vi "Get Properties by Class ID.vi"(8 "error in (no error)":errorcluster, 11 "Class ID":string) -> (0 "error out":errorcluster, 3 "Properties[]":T1(array[cluster]))   [LabVIEW 2023]
doc: "<b> </b> <b> </b>\n© 2017 Q Software Innovations, LLC\nwritten by Quentin \"Q\" Alldredge\nproduced in LabVIEW 2015\n\nsupport@qsoftwareinnovations.com\nwww.qsoftwareinnovations.com\n\nAll rights reserved.\n\nRedistribution and use in source and binary forms, with or without modification, are permitted provided that the following conditions are met:\n\n * Redistributions of source code must retain the above copyright notice, this list of conditions and the following disclaimer.\n * Redistributions in binary form must reproduce the above copyright notice, this list of conditions and the following disclaimer in the documentation and/or other materials provided with the distribution.\n * Neither the name of Q Software Innovations, LLC. nor the names of its contributors may be used to endorse or promote products derived from this software without specific prior written permission.\n\nTHIS SOFTWARE IS PROVIDED BY THE COPYRIGHT HOLDERS AND CONTRIBUTORS \"AS IS\" AND ANY EXPRESS OR IMPLIED WARRANTIES, INCLUDING, BUT NOT LIMITED TO, THE IMPLIED WARRANTIES OF MERCHANTABILITY AND FITNESS FOR A PARTICULAR PURPOSE ARE DISCLAIMED. IN NO EVENT SHALL THE COPYRIGHT OWNER OR CONTRIBUTORS BE LIABLE FOR ANY DIRECT, INDIRECT, INCIDENTAL, SPECIAL, EXEMPLARY, OR CONSEQUENTIAL DAMAGES (INCLUDING, BUT NOT LIMITED TO, PROCUREMENT OF SUBSTITUTE GOODS OR SERVICES; LOSS OF USE, DATA, OR PROFITS; OR BUSINESS INTERRUPTION) HOWEVER CAUSED AND ON ANY THEORY OF LIABILITY, WHETHER IN CONTRACT, STRICT LIABILITY, OR TORT (INCLUDING NEGLIGENCE OR OTHERWISE) ARISING IN ANY WAY OUT OF THE USE OF THIS SOFTWARE, EVEN IF ADVISED OF THE POSSIBILITY OF SUCH DAMAGE."
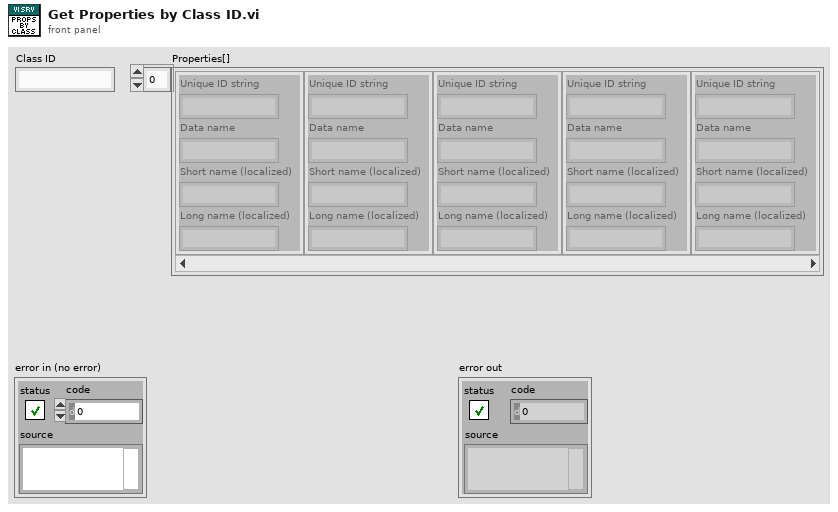
[diagram p1: front panel]
types:
  T1 = cluster{"Unique ID string":string, "Data name":string, "Short name (localized)":string, "Long name (localized)":string}[]
  T2 = typedef "ASPM_ArrayOfUniqueIDStringDatanameShortnameLongname.ctl" = T3[]
  T3 = typedef "ASPM_UniqueIDStringDatanameShortnameLongname.ctl" = cluster{"Unique ID string":string, "Data name":string, "Short name (localized)":string, "Long name (localized)":string}
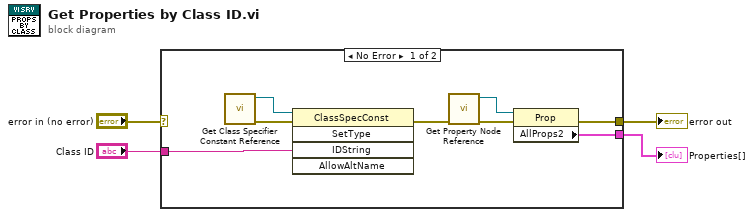
[diagram p0: block diagram]
diagram:
  n1 = case shown="No Error" "error in (no error)" {
    selector: "error in (no error)" -> [_ w13]
    tunnel: [w7 w13] -> w3
    tunnel: "Class ID" -> [w8 _]
    tunnel: [w5 _] -> w1
    frame No Error {
      n2 = call "Get Class Specifier Constant Reference.vi"() -> ("error out"=w10:errorcluster, "specific class reference"=w11:refnum<vi>)  [unwired: 10 in]
      n3 = invoke class="ClassSpecConst" method="SetType"(reference=w11, error in=w10, "IDString"=w8) -> (error out=w9:errorcluster)  [unwired: 2 in, 4 out]
      n4 = call "Get Property Node Reference.vi"("error in (no error)"=w9) -> ("error out"=w12:errorcluster, "Main Prop Refnum"=w6:refnum<vi>)  [unwired: 8 in, 1 out]
      n5 = property class="Prop"(reference=w6, error in=w12) -> (error out=w7:errorcluster, "AllProps2"=w5:T2)  [unwired: 1 out]
    }
    frame Error {
    }
  }
  "error out" <- w3
  "Properties[]" <- w1
